vi "PathPlanner_Trajectory_asWPILibTrajectory.vi"(11 "PathPlannerTrajectory":T6 {"States"."HolonomicAngular\nvelocity Deg/Sec"."SIN" format="%13.4f"; "States"."HolonomicAngular\nvelocity Deg/Sec"."COS" format="%13.4f"; "States"."HolonomicAngular\nvelocity Deg/Sec"."VALUE" format="%13.4f"; "States"."HolonomicRotation"."SIN" format="%13.4f"; "States"."HolonomicRotation"."COS" format="%13.4f"; "States"."HolonomicRotation"."VALUE" format="%13.4f"; "States"."AngularVelocity"."SIN" format="%13.4f"; "States"."AngularVelocity"."COS" format="%13.4f"; "States"."AngularVelocity"."VALUE" format="%13.4f"; "States"."TrajectoryState"."POSE"."ROTATION"."SIN" format="%13.4f"; "States"."TrajectoryState"."POSE"."ROTATION"."COS" format="%13.4f"; "States"."TrajectoryState"."POSE"."ROTATION"."VALUE" format="%13.4f"; "States"."TrajectoryState"."POSE"."TRANSLATION"."Y" format="%14.3f"; "States"."TrajectoryState"."POSE"."TRANSLATION"."X" format="%14.3f"; "States"."AngularAcceleration"."SIN" format="%13.4f"; "States"."AngularAcceleration"."COS" format="%13.4f"; "States"."AngularAcceleration"."VALUE" format="%13.4f"}) -> (3 "TRAJECTORY":T1 {"States"."POSE"."ROTATION"."SIN" format="%13.4f"; "States"."POSE"."ROTATION"."COS" format="%13.4f"; "States"."POSE"."ROTATION"."VALUE" format="%13.4f"; "States"."POSE"."TRANSLATION"."Y" format="%14.3f"; "States"."POSE"."TRANSLATION"."X" format="%14.3f"; "TotalTImeSecs" format="%20.3f"})   [LabVIEW 2019, in "PathPlanner24.lvlib"]
doc: "Convert a PathPlanner trajectory into a LabVIEW / WPILib Trajectory. \n\nInputs:\n -- PathPlannerTrajectory -- PathPlanner Trajectory data cluster\n\nOutputs\n -- Traectory -- LabVIEW traectory library (WPlib style) trajectory data cluster."
uses:
  PathPlanner24.lvlib
  <vilib>/Rock Robotics/WPI/ThirdParty/JAS_Junk/TrajLib/TypeDef/TRANSLATION2D.ctl
  <vilib>/Rock Robotics/WPI/ThirdParty/JAS_Junk/TrajLib/Trajectory_Library.lvlib
  <vilib>/Rock Robotics/WPI/ThirdParty/JAS_Junk/TrajLib/TypeDef/ROTATION2D.ctl
  <vilib>/Rock Robotics/WPI/ThirdParty/JAS_Junk/TrajLib/TypeDef/POSE2D.ctl
  <vilib>/Rock Robotics/WPI/ThirdParty/JAS_Junk/TrajLib/TypeDef/TRAJ_STATE.ctl
  PathPlannerTrajectoryState.ctl
  PathPlannerTrajectory.ctl
  <vilib>/Rock Robotics/WPI/ThirdParty/JAS_Junk/TrajLib/TypeDef/TRAJECTORY.ctl
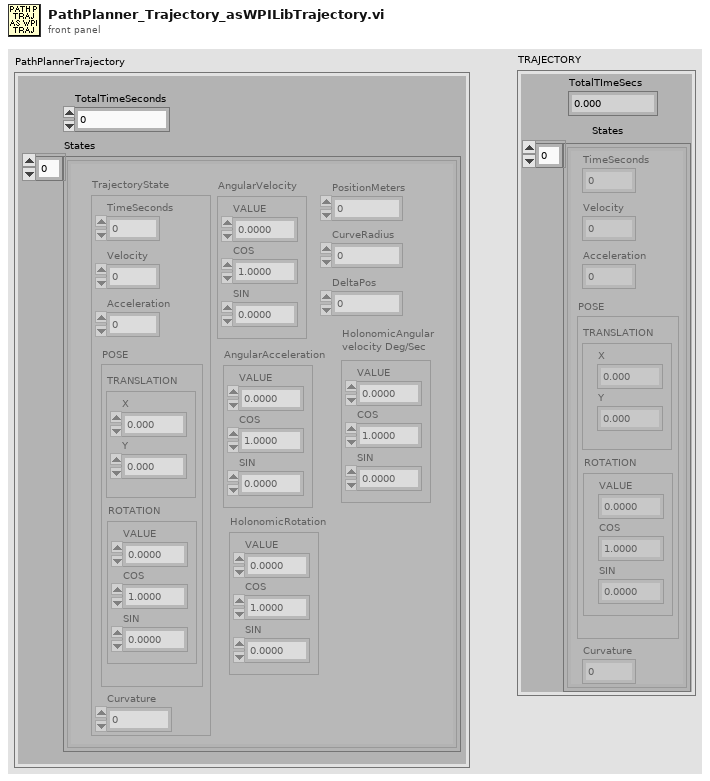
[diagram p1: front panel]
types:
  T1 = typedef "Trajectory_Library.lvlib/TRAJECTORY.ctl" = cluster{"TotalTImeSecs":dbl, "States":T2[]}
  T2 = typedef "Trajectory_Library.lvlib/TRAJ_STATE.ctl" = cluster{"TimeSeconds":dbl, "Velocity":dbl, "Acceleration":dbl, "POSE":T3, "Curvature":dbl}
  T3 = typedef "Trajectory_Library.lvlib/POSE2D.ctl" = cluster{"TRANSLATION":T4, "ROTATION":T5}
  T4 = typedef "Trajectory_Library.lvlib/TRANSLATION2D.ctl" = cluster{"X":dbl, "Y":dbl}
  T5 = typedef "Trajectory_Library.lvlib/ROTATION2D.ctl" = cluster{"VALUE":dbl, "COS":dbl, "SIN":dbl}
  T6 = typedef "PathPlanner24.lvlib/PathPlannerTrajectory.ctl" = cluster{"TotalTimeSeconds":dbl, "States":T7[]}
  T7 = typedef "PathPlanner24.lvlib/PathPlannerTrajectoryState.ctl" = cluster{"AngularAcceleration":T5, "PositionMeters":dbl, "TrajectoryState":T2, "AngularVelocity":T5, "HolonomicRotation":T5, "CurveRadius":dbl, "DeltaPos":dbl, "HolonomicAngular\nvelocity Deg/Sec":T5}
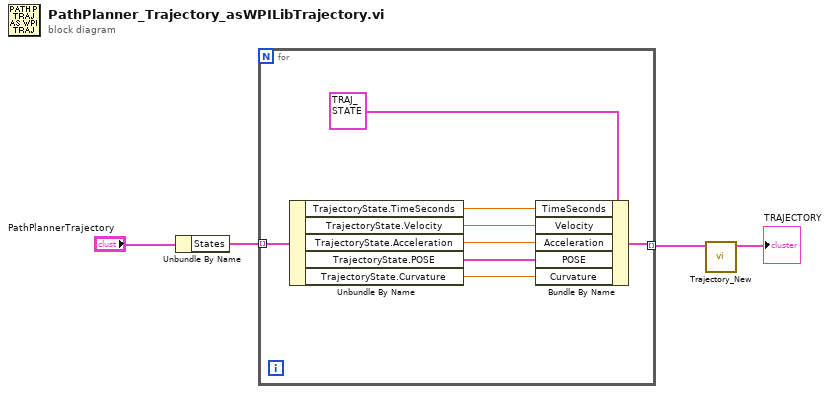
[diagram p0: block diagram]
diagram:
  n1 = Unbundle By Name("PathPlannerTrajectory") -> ("States"=w3:T7[])
  n2 = for {
    tunnel: w3 -> [w12] mode=indexing
    tunnel: [w5] -> w2 mode=indexing
    n3 = Unbundle By Name(w12) -> ("TrajectoryState.TimeSeconds"=w10:dbl, "TrajectoryState.Velocity"=w9:dbl, "TrajectoryState.Acceleration"=w8:dbl, "TrajectoryState.POSE"=w7:T3, "TrajectoryState.Curvature"=w6:dbl)
    n4 = Bundle By Name(cluster=T2 {"TimeSeconds"=0.0, "Velocity"=0.0, "Acceleration"=0.0, "POSE"={"TRANSLATION"={"X"=0.0, "Y"=0.0}, "ROTATION"={"VALUE"=0.0, "COS"=1.0, "SIN"=0.0}}, "Curvature"=0.0} ("TRAJ_STATE"), "TimeSeconds"=w10, "Velocity"=w9, "Acceleration"=w8, "POSE"=w7, "Curvature"=w6) -> (w5:T2)
  }
  n5 = call <vilib>:"Trajectory_New.vi"("TRAJ_STATES"=w2) -> ("TRAJECTORY"=→"TRAJECTORY":T1)  [unwired: 10 in]
